vi "CRYCalc Time Serial Envelope.vi"(4 "dB ref":dbl, 6 "Y data":u16, 7 "Loose part Info":T1 {"Averaging Time" format="%#_6p"}, 8 "FStop":dbl=20.0 min=1.0, 9 "FStart":dbl=1000.0 min=1.0, 10 "Fs":dbl, 11 "Signal In":dbl[](array[numeric])) -> (0 "Loose Particle dT":dbl, 2 "Loose Particle Wave Out":dbl[](array[numeric]), 3 "Loose Particle Envelope Out":dbl[](array[numeric]))   [LabVIEW 2013]
uses:
  <vilib>/Analysis/baseanly.llb/Mean (DBL).vi
  <vilib>/Analysis/5stat.llb/RMS (DBL).vi
  <vilib>/Analysis/baseanly.llb/Unimode.vi
  <vilib>/Analysis/NI_AALBase.lvlib
  <vilib>/Analysis/NI_AALPro.lvlib
  <vilib>/Analysis/3filter.llb/Filter Passband Type.ctl
  <vilib>/Analysis/3filter.llb/Bessel Filter (DBL).vi
  <vilib>/addons/_Advanced Signal Processing/NI_AdvSigProcTSA.lvlib
  <vilib>/addons/Time Series Analysis/Series Preprocess.llb/TSA Exponential Average (Waveform).vi
  <vilib>/Analysis/4window.llb/Cosine Tapered Window (DBL).vi
panel:
  out "min value":dbl
  out "DC estimate (V) 3":dbl format="%0.2f"
  out "DC estimate (V) 2":dbl format="%0.2f"
  out "DC estimate (V)":dbl format="%.6f"
  out "Waveform Graph":dynamicdata(graph)
  in  "Statistic":T2(ring)
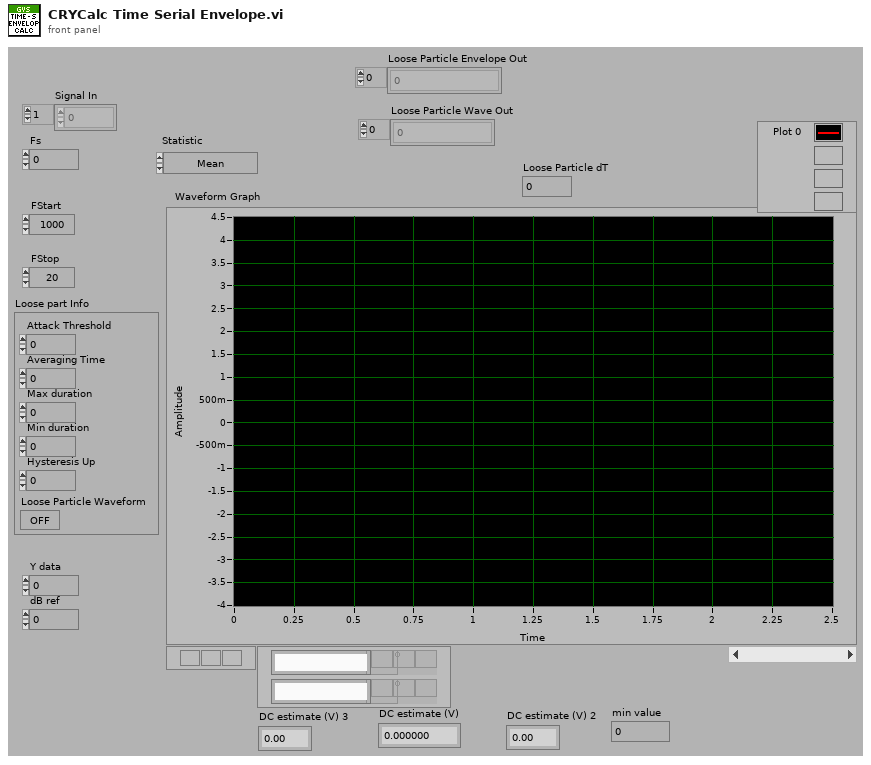
[diagram p1: front panel]
types:
  T1 = cluster{"Attack Threshold":dbl, "Averaging Time":dbl, "Max duration":dbl, "Min duration":dbl, "Hysteresis Up":dbl, "Loose Particle Waveform":bool}
  T2 = enum16{"Mean", "Standard Deviation", "Variance", "Skewness", "Kurtosis", "Median", "Mode", "RMS"}
  T3 = typedef "NI_AALBase.lvlib/Filter Passband Type.ctl" = enum32{"Lowpass", "Highpass", "Bandpass", "Bandstop"}
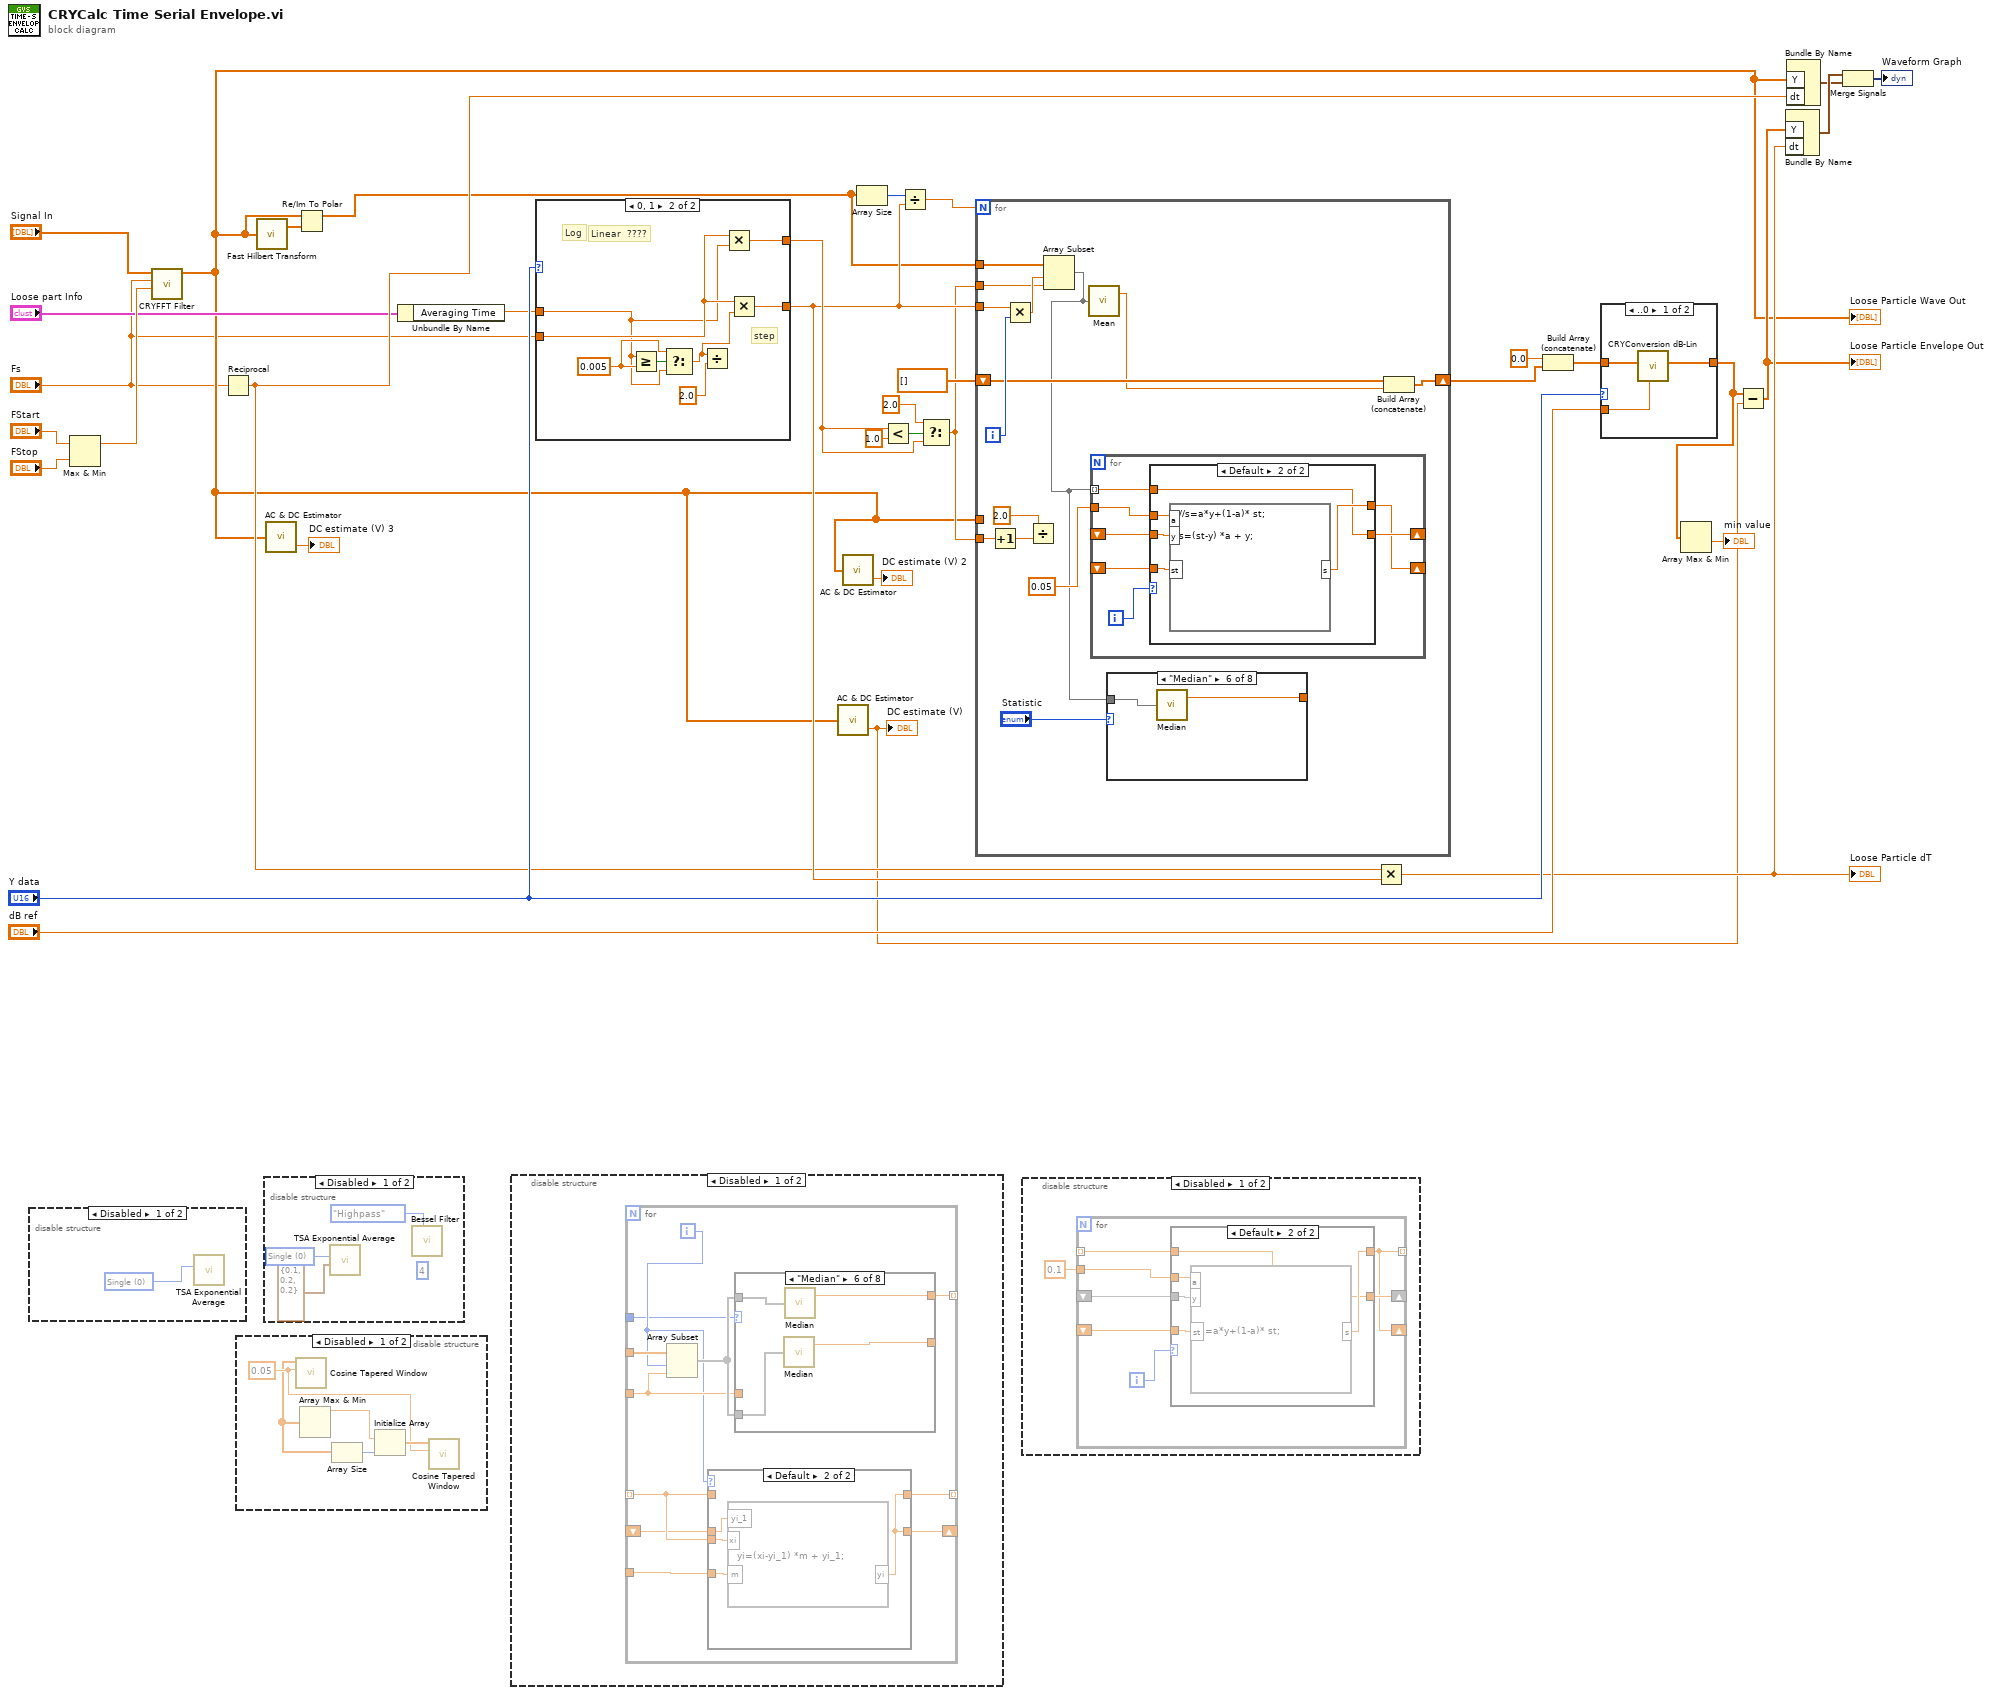
[diagram p0: block diagram]
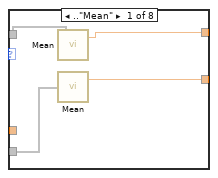
[diagram p3: hidden frame]
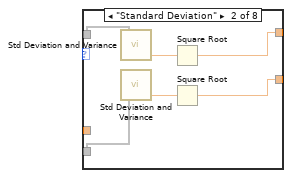
[diagram p4: hidden frame]
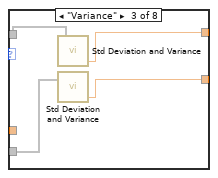
[diagram p5: hidden frame]
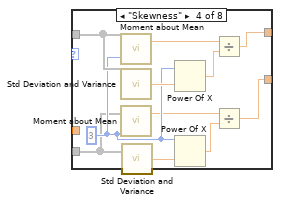
[diagram p6: hidden frame]
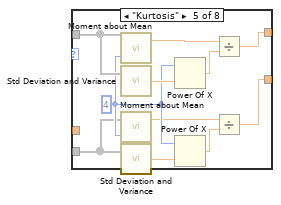
[diagram p7: hidden frame]
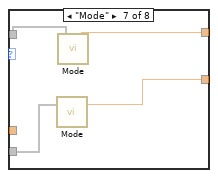
[diagram p8: hidden frame]
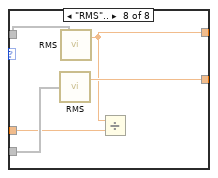
[diagram p9: hidden frame]
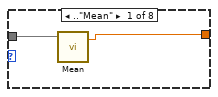
[diagram p15: hidden frame]
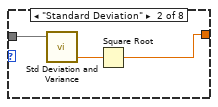
[diagram p16: hidden frame]
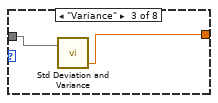
[diagram p17: hidden frame]
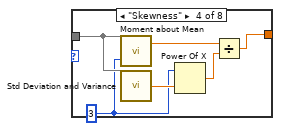
[diagram p18: hidden frame]
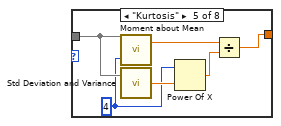
[diagram p19: hidden frame]
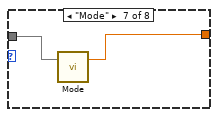
[diagram p20: hidden frame]
diagram:
  n1 = disable-structure shown="Disabled" {
    frame Disabled {
      w36 = u16 0 items=["Single", "Double", "Triple"] ("exponential type")
      n2 = call-poly <vilib>:"TSA Exponential Average.vi"("exponential type"=w36) -> ("Xt"=w37:waveform(dbl))  [unwired: 8 in, 2 out]
    }
    frame Enabled {
    }
  }
  n3 = Max & Min(x="FStart", y="FStop") -> (max(x,y)=w32:dbl)  [unwired: 1 out]
  n4 = call "CRYFFT Filter.vi"("Cutoff Freq"=w32, "Fs"="Fs", "Signal In"="Signal In") -> ("Signal out"=w3:dbl[])  [unwired: 8 in]
  "Loose Particle Wave Out" <- w3
  n5 = Reciprocal(x="Fs") -> (1/x=w17:dbl)
  n6 = disable-structure shown="Disabled" {
    frame Disabled {
      w39 = 0.05 ("ratio")
      n7 = Array Max & Min() -> (array=w38:dbl[], max value=w40:dbl)  [unwired: 3 out]
      n8 = call-poly <vilib>:"Cosine Tapered Window.vi"("ratio"=w39, "X"=w38) -> ()  [unwired: 8 in, 2 out]
      n9 = Array Size(array=w38) -> (size(s)=w42:i32)
      n10 = Initialize Array(w40, w42) -> (w41:dbl[])
      n11 = call-poly <vilib>:"Cosine Tapered Window.vi"("ratio"=w39, "X"=w41) -> ()  [unwired: 8 in, 2 out]
    }
    frame Enabled {
    }
  }
  n12 = call <vilib>:"Fast Hilbert Transform.vi"("X"=w3) -> ("Hilbert{X}"=w35:dbl[])  [unwired: 1 out]
  n13 = disable-structure shown="Disabled" {
    frame Disabled {
      w43 = u16 0 items=["Single", "Double", "Triple"] ("exponential type")
      (unwired) 4 ("order")
      n14 = call-poly <vilib>:"TSA Exponential Average.vi"("exponential factors"=cluster{"level":dbl, "trend":dbl, "season":dbl} {"level"=0.1, "trend"=0.2, "season"=0.2}, "exponential type"=w43) -> ()  [unwired: 8 in, 2 out]
      n15 = call-poly <vilib>:"Bessel Filter.vi"("filter type"=Filter_Passband_Type."Highpass") -> ()  [unwired: 7 in, 2 out]
    }
    frame Enabled {
    }
  }
  n16 = call <vilib>:"AC & DC Estimator.vi"("Signal (V)"=w3) -> ("DC estimate (V)"=→"DC estimate (V) 3":dbl)  [unwired: 1 out]
  n17 = Re/Im To Polar(2:w35, 3:w3) -> (1:w7:dbl[])  [unwired: 1 out]
  n18 = Unbundle By Name("Loose part Info") -> ("Averaging Time"=w13:dbl)
  n19 = disable-structure shown="Disabled" {
    frame Disabled {
      n20 = for {
        tunnel: _ -> [w57]
        tunnel: [w55] -> _ mode=indexing
        tunnel: _ -> [w54]
        tunnel: _ -> [w52]
        tunnel: [w53] -> _ mode=indexing
        tunnel: _ -> [w51] mode=indexing
        shift-right: [w50] -> _
        shift-left: _ -> [w49]
        tunnel: [w47] -> w46
        i -> [w48]
        n21 = Array Subset(array=w57, index=w48, length=w54) -> (w56:void[])
        n22 = case shown="Default" w48 {
          tunnel: w51 -> [w58 _]
          tunnel: [w58 w60] -> w53
          tunnel: w52 -> [_ w62]
          tunnel: w51 -> [_ w61]
          tunnel: [w58 w60] -> w50
          tunnel: w49 -> [_ w59]
          frame 0 {
          }
          frame Default {
            n23 = formula code="yi=(xi-yi_1) *m + yi_1;"("m"=w62, "xi"=w61, "yi_1"=w59) -> ("yi"=w60:dbl)
          }
        }
        n24 = case shown="\"Median\"" w47 {
          tunnel: w56 -> [w66 w71 w75 w82 w93 w102 w106 w111]
          tunnel: [w64 w68 w74 w79 w90 w100 w104 w110] -> _
          tunnel: [w65 w72 w76 w83 w94 w101 w105 w107] -> w55
          tunnel: w56 -> [w63 w67 w73 w86 w97 w99 w103 w109]
          tunnel: w54 -> [_ _ _ _ _ _ _ w108]
          frame .."Mean" {
            n25 = call-poly <vilib>:"Mean.vi"("X"=w63) -> ("mean"=w65:dbl)  [unwired: 1 out]
            n26 = call-poly <vilib>:"Mean.vi"("X"=w66) -> ("mean"=w64:dbl)  [unwired: 1 out]
          }
          frame "Standard Deviation" {
            n27 = call <vilib>:"Std Deviation and Variance.vi"("X"=w67) -> ("variance"=w70:dbl)  [unwired: 1 in, 2 out]
            n28 = call <vilib>:"Std Deviation and Variance.vi"("X"=w71) -> ("variance"=w69:dbl)  [unwired: 1 in, 2 out]
            n29 = Square Root(x=w70) -> (sqrt(x)=w72:dbl)
            n30 = Square Root(x=w69) -> (sqrt(x)=w68:dbl)
          }
          frame "Variance" {
            n31 = call <vilib>:"Std Deviation and Variance.vi"("X"=w73) -> ("variance"=w76:dbl)  [unwired: 1 in, 2 out]
            n32 = call <vilib>:"Std Deviation and Variance.vi"("X"=w75) -> ("variance"=w74:dbl)  [unwired: 1 in, 2 out]
          }
          frame "Skewness" {
            w84 = 3
            n33 = call <vilib>:"Moment about Mean.vi"("order"=w84, "X"=w86) -> ("moment"=w77:dbl)  [unwired: 1 out]
            n34 = call <vilib>:"Std Deviation and Variance.vi"("X"=w86) -> ("standard deviation"=w87:dbl)  [unwired: 1 in, 2 out]
            n35 = call <vilib>:"Moment about Mean.vi"("order"=w84, "X"=w82) -> ("moment"=w80:dbl)  [unwired: 1 out]
            n36 = call <vilib>:"Std Deviation and Variance.vi"("X"=w82) -> ("standard deviation"=w85:dbl)  [unwired: 1 in, 2 out]
            n37 = Power Of X(1:w87, 2:w84) -> (0:w78:dbl)
            n38 = Power Of X(1:w85, 2:w84) -> (0:w81:dbl)
            n39 = Divide(x=w77, y=w78) -> (x/y=w83:dbl)
            n40 = Divide(x=w80, y=w81) -> (x/y=w79:dbl)
          }
          frame "Kurtosis" {
            w95 = 4
            n41 = call <vilib>:"Moment about Mean.vi"("order"=w95, "X"=w97) -> ("moment"=w89:dbl)  [unwired: 1 out]
            n42 = call <vilib>:"Std Deviation and Variance.vi"("X"=w97) -> ("standard deviation"=w98:dbl)  [unwired: 1 in, 2 out]
            n43 = call <vilib>:"Moment about Mean.vi"("order"=w95, "X"=w93) -> ("moment"=w91:dbl)  [unwired: 1 out]
            n44 = call <vilib>:"Std Deviation and Variance.vi"("X"=w93) -> ("standard deviation"=w96:dbl)  [unwired: 1 in, 2 out]
            n45 = Power Of X(1:w98, 2:w95) -> (0:w88:dbl)
            n46 = Power Of X(1:w96, 2:w95) -> (0:w92:dbl)
            n47 = Divide(x=w89, y=w88) -> (x/y=w94:dbl)
            n48 = Divide(x=w91, y=w92) -> (x/y=w90:dbl)
          }
          frame "Median" {
            n49 = call <vilib>:"Median.vi"("X"=w102) -> ("median"=w100:dbl)  [unwired: 1 out]
            n50 = call <vilib>:"Median.vi"("X"=w99) -> ("median"=w101:dbl)  [unwired: 1 out]
          }
          frame "Mode" {
            n51 = call-poly <vilib>:"Mode.vi"("X"=w106) -> ("mode"=w104:dbl)  [unwired: 1 in, 1 out]
            n52 = call-poly <vilib>:"Mode.vi"("X"=w103) -> ("mode"=w105:dbl)  [unwired: 1 in, 1 out]
          }
          frame "RMS".. {
            n53 = call-poly <vilib>:"RMS.vi"("X"=w111) -> ("rms value"=w110:dbl)  [unwired: 1 out]
            n54 = call-poly <vilib>:"RMS.vi"("X"=w109) -> ("rms value"=w107:dbl)  [unwired: 1 out]
            n55 = Divide(x=w107, y=w108) -> ()  [unwired: 1 out]
          }
        }
      }
    }
    frame Enabled {
    }
  }
  n56 = case shown="0, 1" "Y data" {
    tunnel: "Fs" -> [w114 w118]
    tunnel: [w113 w122] -> w21
    tunnel: [w113 w117] -> w23
    tunnel: w13 -> [w112 w116]
    frame Default {
      n57 = Multiply(x=w114, y=w112) -> (x*y=w113:dbl)
    }
    frame 0, 1 {
      w120 = 0.005 ("y")
      # "Log"
      # "Linear  ????"
      # "step"
      n58 = Greater Or Equal?(x=w116, y=w120) -> (x >= y?=w121:bool)
      n59 = Select(t=w120, s=w121, f=w116) -> (s? t:f=w115:dbl)
      n60 = Divide(x=w115, y=2.0) -> ()  [unwired: 1 out]
      n61 = Multiply(x=w118, y=w116) -> (x*y=w117:dbl)
      n62 = Multiply(x=w118, y=w115) -> (x*y=w122:dbl)
    }
  }
  n63 = call <vilib>:"AC & DC Estimator.vi"("Signal (V)"=w3) -> ("DC estimate (V)"=w11:dbl)  [unwired: 1 out]
  "DC estimate (V)" <- w11
  n64 = call <vilib>:"AC & DC Estimator.vi"("Signal (V)"=w3) -> ("DC estimate (V)"=→"DC estimate (V) 2":dbl)  [unwired: 1 out]
  n65 = Array Size(array=w7) -> (size(s)=w28:i32)
  n66 = Less?(x=w23, y=1.0) -> (x < y?=w26:bool)
  n67 = Divide(x=w28, y=w21) -> (x/y=w27:dbl)
  n68 = Select(t=2.0, s=w26, f=w23) -> (s? t:f=w8:dbl)
  n69 = for {
    N: w27 -> [_]
    tunnel: w7 -> [w124]
    tunnel: w8 -> [w134]
    shift-right: [w131] -> w5
    shift-left: dbl[] [] ("Ramp Pattern") -> [w132]
    tunnel: w21 -> [w133]
    tunnel: w3 -> [_]
    tunnel: w8 -> [w130]
    i -> [w135]
    n70 = Increment(x=w130) -> (x+1=w128:dbl)
    n71 = Multiply(x=w133, y=w135) -> (x*y=w136:dbl)
    n72 = Divide(x=2.0, y=w128) -> ()  [unwired: 1 out]
    n73 = Array Subset(array=w124, index=w136, length=w134) -> (w126:dbl[])
    n74 = call-poly <vilib>:"Mean.vi"("X"=w126) -> ("mean"=w123:dbl)  [unwired: 1 out]
    n75 = for {
      tunnel: w126 -> [w168] mode=indexing
      shift-right: [w164] -> _
      shift-left: _ -> [w165]
      tunnel: 0.05 ("rms value") -> [w167]
      shift-right: [w162] -> _
      shift-left: _ -> [w166]
      i -> [w163]
      n76 = case shown="Default" w163 {
        tunnel: w168 -> [w169 w170]
        tunnel: [w169 w172] -> w162
        tunnel: w166 -> [_ w174]
        tunnel: w167 -> [_ w173]
        tunnel: w165 -> [_ w171]
        tunnel: [w169 w170] -> w164
        frame 0 {
        }
        frame Default {
          n77 = formula code="//s=a*y+(1-a)* st;\n\ns=(st-y) *a + y;"("st"=w174, "a"=w173, "y"=w171) -> ("s"=w172:dbl)
        }
      }
    }
    n78 = case shown="\"Median\"" "Statistic" {
      tunnel: [w138 w141 w143 w146 w152 w157 w159 w160] -> _
      tunnel: w126 -> [w137 w139 w142 w148 w154 w156 w158 w161]
      frame .."Mean" {
        n79 = call-poly <vilib>:"Mean.vi"("X"=w137) -> ("mean"=w138:dbl)  [unwired: 1 out]
      }
      frame "Standard Deviation" {
        n80 = call <vilib>:"Std Deviation and Variance.vi"("X"=w139) -> ("variance"=w140:dbl)  [unwired: 1 in, 2 out]
        n81 = Square Root(x=w140) -> (sqrt(x)=w141:dbl)
      }
      frame "Variance" {
        n82 = call <vilib>:"Std Deviation and Variance.vi"("X"=w142) -> ("variance"=w143:dbl)  [unwired: 1 in, 2 out]
      }
      frame "Skewness" {
        w147 = 3
        n83 = call <vilib>:"Moment about Mean.vi"("order"=w147, "X"=w148) -> ("moment"=w144:dbl)  [unwired: 1 out]
        n84 = call <vilib>:"Std Deviation and Variance.vi"("X"=w148) -> ("standard deviation"=w149:dbl)  [unwired: 1 in, 2 out]
        n85 = Power Of X(1:w149, 2:w147) -> (0:w145:dbl)
        n86 = Divide(x=w144, y=w145) -> (x/y=w146:dbl)
      }
      frame "Kurtosis" {
        w153 = 4
        n87 = call <vilib>:"Moment about Mean.vi"("order"=w153, "X"=w154) -> ("moment"=w151:dbl)  [unwired: 1 out]
        n88 = call <vilib>:"Std Deviation and Variance.vi"("X"=w154) -> ("standard deviation"=w155:dbl)  [unwired: 1 in, 2 out]
        n89 = Power Of X(1:w155, 2:w153) -> (0:w150:dbl)
        n90 = Divide(x=w151, y=w150) -> (x/y=w152:dbl)
      }
      frame "Median" {
        n91 = call <vilib>:"Median.vi"("X"=w156) -> ("median"=w157:dbl)  [unwired: 1 out]
      }
      frame "Mode" {
        n92 = call-poly <vilib>:"Mode.vi"("X"=w158) -> ("mode"=w159:dbl)  [unwired: 1 in, 1 out]
      }
      frame "RMS".. {
        n93 = call-poly <vilib>:"RMS.vi"("X"=w161) -> ("rms value"=w160:dbl)  [unwired: 1 out]
      }
    }
    n94 = Build Array (concatenate)(w132, w123) -> (w131:dbl[])
  }
  n95 = disable-structure shown="Disabled" {
    frame Disabled {
      n96 = for {
        tunnel: _ -> [w182] mode=indexing
        tunnel: [w176] -> _ mode=indexing
        shift-right: [w178] -> _
        shift-left: _ -> [w179]
        tunnel: 0.1 ("rms value") -> [w181]
        shift-right: [w176] -> _
        shift-left: _ -> [w180]
        i -> [w177]
        n97 = case shown="Default" w177 {
          tunnel: w182 -> [w183 w184]
          tunnel: [w183 w186] -> w176
          tunnel: w180 -> [_ w188]
          tunnel: w181 -> [_ w187]
          tunnel: w179 -> [_ w185]
          tunnel: [w183 w184] -> w178
          frame 0 {
          }
          frame Default {
            n98 = formula code="s=a*y+(1-a)* st;"("st"=w188, "a"=w187, "y"=w185) -> ("s"=w186:dbl)
          }
        }
      }
    }
    frame Enabled {
    }
  }
  n99 = Multiply(x=w17, y=w21) -> (x*y=w20:dbl)
  "Loose Particle dT" <- w20
  n100 = Build Array (concatenate)(0.0 ("element"), w5) -> (w16:dbl[])
  n101 = case shown="..0" "Y data" {
    tunnel: w16 -> [w191 w192]
    tunnel: "dB ref" -> [w189 _]
    tunnel: [w190 w192] -> w4
    frame ..0 {
      n102 = call "CRYConversion dB-Lin.vi"("dB ref."=w189, "Lin In array"=w191) -> ("Log Out array"=w190:dbl[])  [unwired: 4 in, 3 out]
    }
    frame 1.. {
    }
  }
  n103 = Array Max & Min(array=w4) -> (min value=→"min value":dbl)  [unwired: 3 out]
  n104 = Subtract(x=w4, y=w11) -> (x-y=w6:dbl[])
  "Loose Particle Envelope Out" <- w6
  n105 = Bundle By Name("Y"=w6, "dt"=w20) -> (w19:waveform(dbl))  [unwired: 1 in]
  n106 = Bundle By Name("Y"=w3, "dt"=w17) -> (w18:waveform(dbl))  [unwired: 1 in]
  n107 = Merge Signals(w19, w18) -> (→"Waveform Graph":dynamicdata)
